vi "Waveform to Cluster.vi"(8 "Error In":errorcluster, 9 "Input":waveform(dbl)[](array[waveform]), 10 "Input String":string) -> (0 "Error Out":errorcluster, 1 "Output":cluster{"Y":dbl[]}[](array[cluster]), 2 "Output Label":string[](array[string]))   [LabVIEW 2019, in "SMO.Transport.lvclass"]
uses:
  SMO.Transport.lvclass
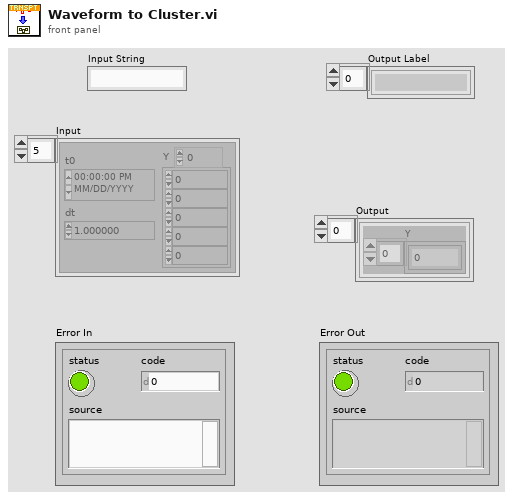
[diagram p1: front panel]
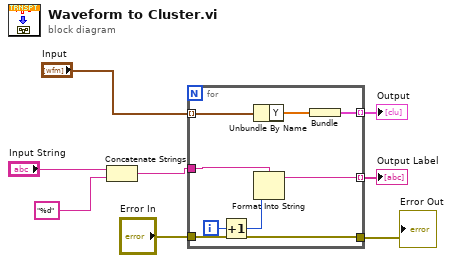
[diagram p0: block diagram]
diagram:
  n1 = Concatenate Strings("Input String", "%d" ("wavenames")) -> (w6:string)
  n2 = for {
    tunnel: [w15] -> w4 mode=indexing
    tunnel: [w13] -> w5 mode=indexing
    tunnel: w6 -> [w11]
    tunnel: "Input" -> [w10] mode=indexing
    tunnel: "Error In" -> [w9]
    tunnel: [w9] -> w2
    i -> [w16]
    n3 = Increment(x=w16) -> (x+1=w14:i32)
    n4 = Unbundle By Name(w10) -> ("Y"=w12:dbl[])
    n5 = Format Into String(format string=w11, w14) -> (resulting string=w15:string)  [unwired: 2 in, 1 out]
    n6 = Bundle("Y"=w12) -> (w13:cluster{"Y":dbl[]})  [unwired: 1 in]
  }
  "Output" <- w5
  "Output Label" <- w4
  "Error Out" <- w2
